vi "Do_Move_tl.vi"(2 "CHANNEL PARAMETERS":string[][](table), 4 "Abs Pos REQD.":dbl step=0.00125 format="%.5f", 5 "Axis Name":string) -> (0 "Move OK?":bool, 1 "Abs Pos ACHVD.":dbl format="%.5f")   [LabVIEW 2010]
uses:
  Traverse_setup_tl.glob.vi
panel:
  in  "Case Constant\n(See Context Help)":bool=TRUE
  out "PRO-J TARGET pos":i32
  out "PRO-J start pos":i32
  out "PULSES/mm":dbl format="%.2f"
  out "PRO-J MOVE LENGTH":i32
  out "Mac start pos":dbl format="%.5f"
  out "PRO-J Final Pos":i32
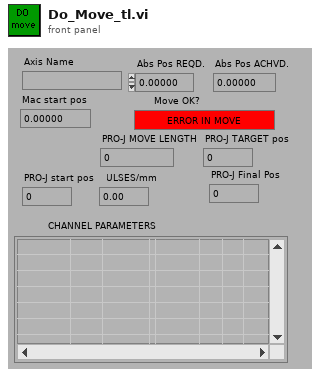
[diagram p1: front panel]
types:
  T1 = enum16{"Is Axis Current axis?", "Write Parameters", "Set Address", "Selected OK?", "Update current axis"}
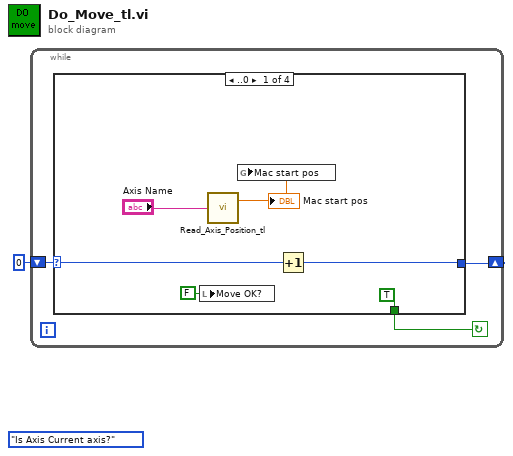
[diagram p0: block diagram]
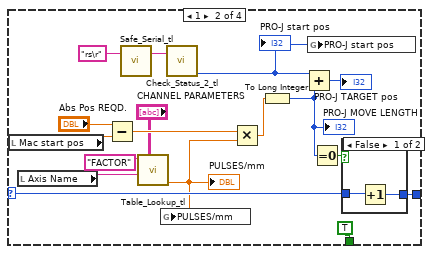
[diagram p2: hidden frame]
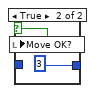
[diagram p3: hidden frame]
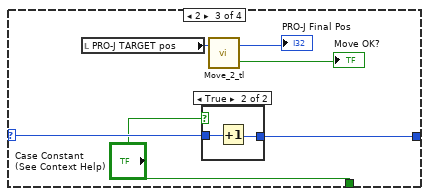
[diagram p4: hidden frame]
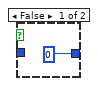
[diagram p5: hidden frame]
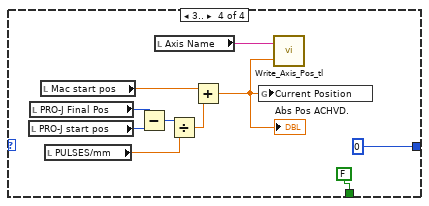
[diagram p6: hidden frame]
diagram:
  (unwired) T1."Is Axis Current axis?"
  n1 = while {
    shift-left: 0 -> [w4]
    shift-right: [w3] -> _
    stop <- w2 continue-if-true
    n2 = case shown="..0" w4 {
      selector: w4 -> [w10 w14 w37 _]
      tunnel: [w7 w27 w36 0] -> w3
      tunnel: [TRUE TRUE "Case Constant\n(See Context Help)" FALSE] -> w2
      frame ..0 {
        n3 = local write "Move OK?"(FALSE) -> ()
        n4 = call "Read_Axis_Position_tl.vi"("Axis"="Axis Name") -> ("Position"=w5:dbl)  [unwired: 1 out]
        "Mac start pos" <- w5
        n5 = global write "Traverse_setup_tl.glob.vi" "Mac start pos"(w5) -> ()
        n6 = Increment(x=w10) -> (x+1=w7:i32)
      }
      frame 1 {
        n7 = local read "Mac start pos"() -> (w22:dbl)
        n8 = local read "Axis Name"() -> (w21:string)
        n9 = Subtract(x="Abs Pos REQD.", y=w22) -> (x-y=w19:dbl)
        n10 = call "Safe_Serial_tl.vi"("Tx String"="rs\r") -> ("Rx String"=w24:string)  [unwired: 5 in, 1 out]
        n11 = call "Table_Lookup_tl.vi"("Lookup Table"="CHANNEL PARAMETERS", "Search String"=w21, "Required variable"="FACTOR") -> ("Floating Output"=w12:dbl)  [unwired: 1 in, 4 out]
        "PULSES/mm" <- w12
        n12 = global write "Traverse_setup_tl.glob.vi" "PULSES/mm"(w12) -> ()
        n13 = call "Check_Status_2_tl.vi"("Status Request Reply"=w24) -> ("Current Position"=w11:i32)  [unwired: 4 out]
        "PRO-J start pos" <- w11
        n14 = Multiply(x=w19, y=w12) -> (x*y=w18:dbl)
        n15 = To Long Integer(number=w18) -> (32bit integer=w16:i32)
        "PRO-J MOVE LENGTH" <- w16
        n16 = Add(x=w11, y=w16) -> (x+y=→"PRO-J TARGET pos":i32)
        n17 = global write "Traverse_setup_tl.glob.vi" "PRO-J start pos"(w11) -> ()
        n18 = Equal To 0?(x=w16) -> (x = 0?=w15:bool)
        n19 = case shown="False" w15 {
          selector: w15 -> [_ w30]
          tunnel: [w29 3] -> w27
          tunnel: w14 -> [w28 _]
          frame False {
            n20 = Increment(x=w28) -> (x+1=w29:i32)
          }
          frame True {
            n21 = local write "Move OK?"(w30) -> ()
          }
        }
      }
      frame 2 {
        n22 = local read "PRO-J TARGET pos"() -> (w35:i32)
        n23 = case shown="True" "Case Constant\n(See Context Help)" {
          tunnel: w37 -> [_ w40]
          tunnel: [0 w39] -> w36
          frame False {
          }
          frame True {
            n24 = Increment(x=w40) -> (x+1=w39:i32)
          }
        }
        n25 = call "Move_2_tl.vi"("Target Position"=w35) -> ("Move OK?"=→"Move OK?":bool, "Current Position"=→"PRO-J Final Pos":i32)  [unwired: 1 out]
      }
      frame 3.. {
        n26 = local read "PRO-J start pos"() -> (w44:i32)
        n27 = local read "PRO-J Final Pos"() -> (w43:i32)
        n28 = local read "Mac start pos"() -> (w46:dbl)
        n29 = local read "PULSES/mm"() -> (w48:dbl)
        n30 = Subtract(x=w43, y=w44) -> (x-y=w47:i32)
        n31 = local read "Axis Name"() -> (w41:string)
        n32 = Divide(x=w47, y=w48) -> (x/y=w45:dbl)
        n33 = Add(x=w46, y=w45) -> (x+y=w42:dbl)
        "Abs Pos ACHVD." <- w42
        n34 = global write "Traverse_setup_tl.glob.vi" "Current Position"(w42) -> ()
        n35 = call "Write_Axis_Pos_tl.vi"("Position"=w42, "Axis"=w41) -> ()  [unwired: 2 out]
      }
    }
  }
